vi "FindTag__slk_tc.vi"(0 "tree control in":refnum<class "TreeControl.lvclass">, 5 "input text":string, 11 "error in (no error)":errorcluster, 12 "column # (0)":i32) -> (4 "tree control out":refnum<class "TreeControl.lvclass">, 6 "duplicated text":string, 10 "tags":string[](array[string]), 15 "error out":errorcluster)   [LabVIEW 2020, in "TreeControl.lvclass"]
doc: "Searches the tree for tags whose text matches the Input text."
uses:
  Library/TreeControl.lvclass
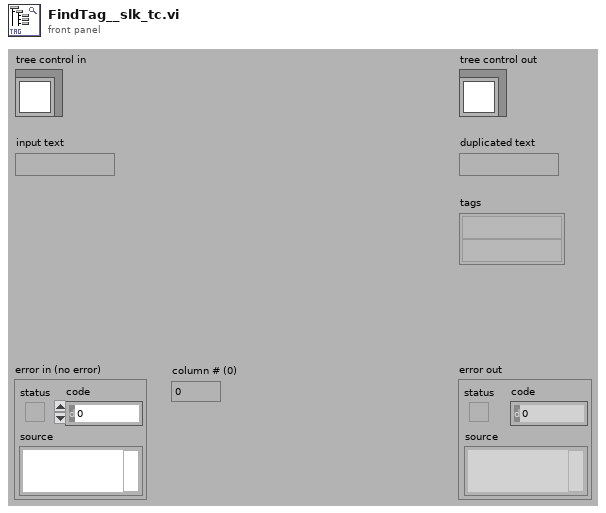
[diagram p1: front panel]
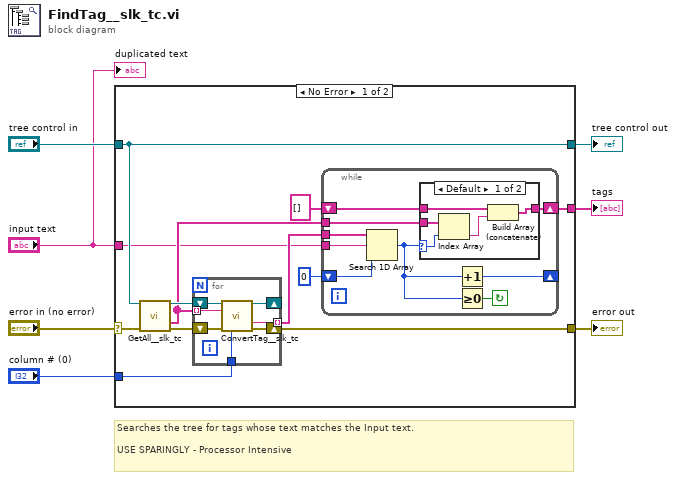
[diagram p0: block diagram]
diagram:
  # "Searches the tree for tags whose text matches the Input text.\n \nUSE SPARINGLY - Processor Intensive"
  n1 = case shown="No Error" "error in (no error)" {
    selector: "error in (no error)" -> [w15 w43]
    tunnel: [w8 w43] -> w6
    tunnel: [w18 w42] -> w4
    tunnel: "tree control in" -> [w18 w42]
    tunnel: "input text" -> [w10 _]
    tunnel: "column # (0)" -> [w16 _]
    tunnel: [w9 _] -> w2
    frame No Error {
      n2 = call "GetAll__slk_tc.vi"("tree control in"=w18, "error in (no error)"=w15) -> ("tree control out"=w19:refnum<class "TreeControl.lvclass">, "output tree items"=w11:string[], "error out"=w17:errorcluster)  [unwired: 11 out]
      n3 = for {
        shift-right: [w39] -> _
        shift-left: w19 -> [w41]
        tunnel: w11 -> [w38] mode=indexing
        shift-right: [w37] -> w8
        shift-left: w17 -> [w40]
        tunnel: [w36] -> w12 mode=indexing
        tunnel: w16 -> [w35]
        n4 = call "ConvertTag__slk_tc.vi"("tree control in"=w41, "input tag (current tag)"=w38, "error in (no error)"=w40, "column # (0)"=w35) -> ("tree control out"=w39:refnum<class "TreeControl.lvclass">, "text"=w36:string, "error out"=w37:errorcluster)  [unwired: 9 out]
      }
      n5 = while {
        tunnel: w12 -> [w28]
        tunnel: w10 -> [w27]
        shift-right: [w25] -> _
        shift-left: 0 ("Start Index (0)") -> [w26]
        shift-right: [w22] -> w9
        shift-left: string[] [] ("Tags") -> [w23]
        tunnel: w11 -> [w20]
        stop <- w21 continue-if-true
        n6 = Search 1D Array(1D array=w28, element=w27, start index (0)=w26) -> (index of element=w24:i32)
        n7 = case shown="Default" w24 {
          selector: w24 -> [w33 _]
          tunnel: w23 -> [w32 w34]
          tunnel: [w31 w34] -> w22
          tunnel: w20 -> [w29 _]
          frame Default {
            n8 = Index Array(array=w29, index=w33) -> (element=w30:string)
            n9 = Build Array (concatenate)(w32, w30) -> (w31:string[])
          }
          frame -1 {
          }
        }
        n10 = Increment(x=w24) -> (x+1=w25:i32)
        n11 = Greater Or Equal To 0?(x=w24) -> (x >= 0?=w21:bool)
      }
    }
    frame Error {
    }
  }
  "error out" <- w6
  "tree control out" <- w4
  "tags" <- w2
  "duplicated text" <- "input text"
